vi "Phsae_shift_test(3).vi"() -> ()   [LabVIEW 2017]
uses:
  <vilib>/Analysis/3filter.llb/Filter Passband Type.ctl
  <vilib>/Analysis/3filter.llb/FIR Windowed Filter (DBL).vi
  <vilib>/measure/maspectr.llb/FFT Spectrum (Real-Im) for 1 Chan.vi
  <vilib>/Analysis/NI_AALBase.lvlib
  <vilib>/Analysis/NI_AALPro.lvlib
  <vilib>/measure/NI_MAPro.lvlib
panel:
  out "최대값":dbl
  out "크기":i32
  out "S3 phase spectrum":waveform(dbl)(graph)
  out "SUM signal":waveform(dbl)(graph)
  out "S3 signal":waveform(dbl)(graph)
  out "S2 signal":waveform(dbl)(graph)
  out "S1 signal":waveform(dbl)(graph)
  out "S0 signal":waveform(dbl)(graph)
  out "S3 FFT":waveform(dbl)(graph)
  out "S2 FFT":waveform(dbl)(graph)
  out "S1 FFT":waveform(dbl)(graph)
  out "S0 FFT":waveform(dbl)(graph)
  in  "S3 Carrier Phsae":dbl=270.0
  in  "S2 Carrier Phsae":dbl=180.0
  in  "S1 Carrier Phsae":dbl=90.0
  in  "S0 Carrier Phsae":dbl=90.0
  in  "S3 Phsae":dbl=270.0
  in  "S2 Phsae":dbl=180.0
  in  "S1 Phsae":dbl=90.0
  in  "S0 Phsae":dbl=90.0
  in  "Carrier Frequency(Hz)":dbl=560000.0
  in  "Frequency(Hz)":dbl=600000.0
  in  "Amplitude(Vpeak)":dbl=1.0
  in  "Pulse length(sec)":dbl=0.5
  in  "Sampling frequency(Hz)":dbl=3000000.0
  in  "Delay time.A.1(sec)":dbl=0.5
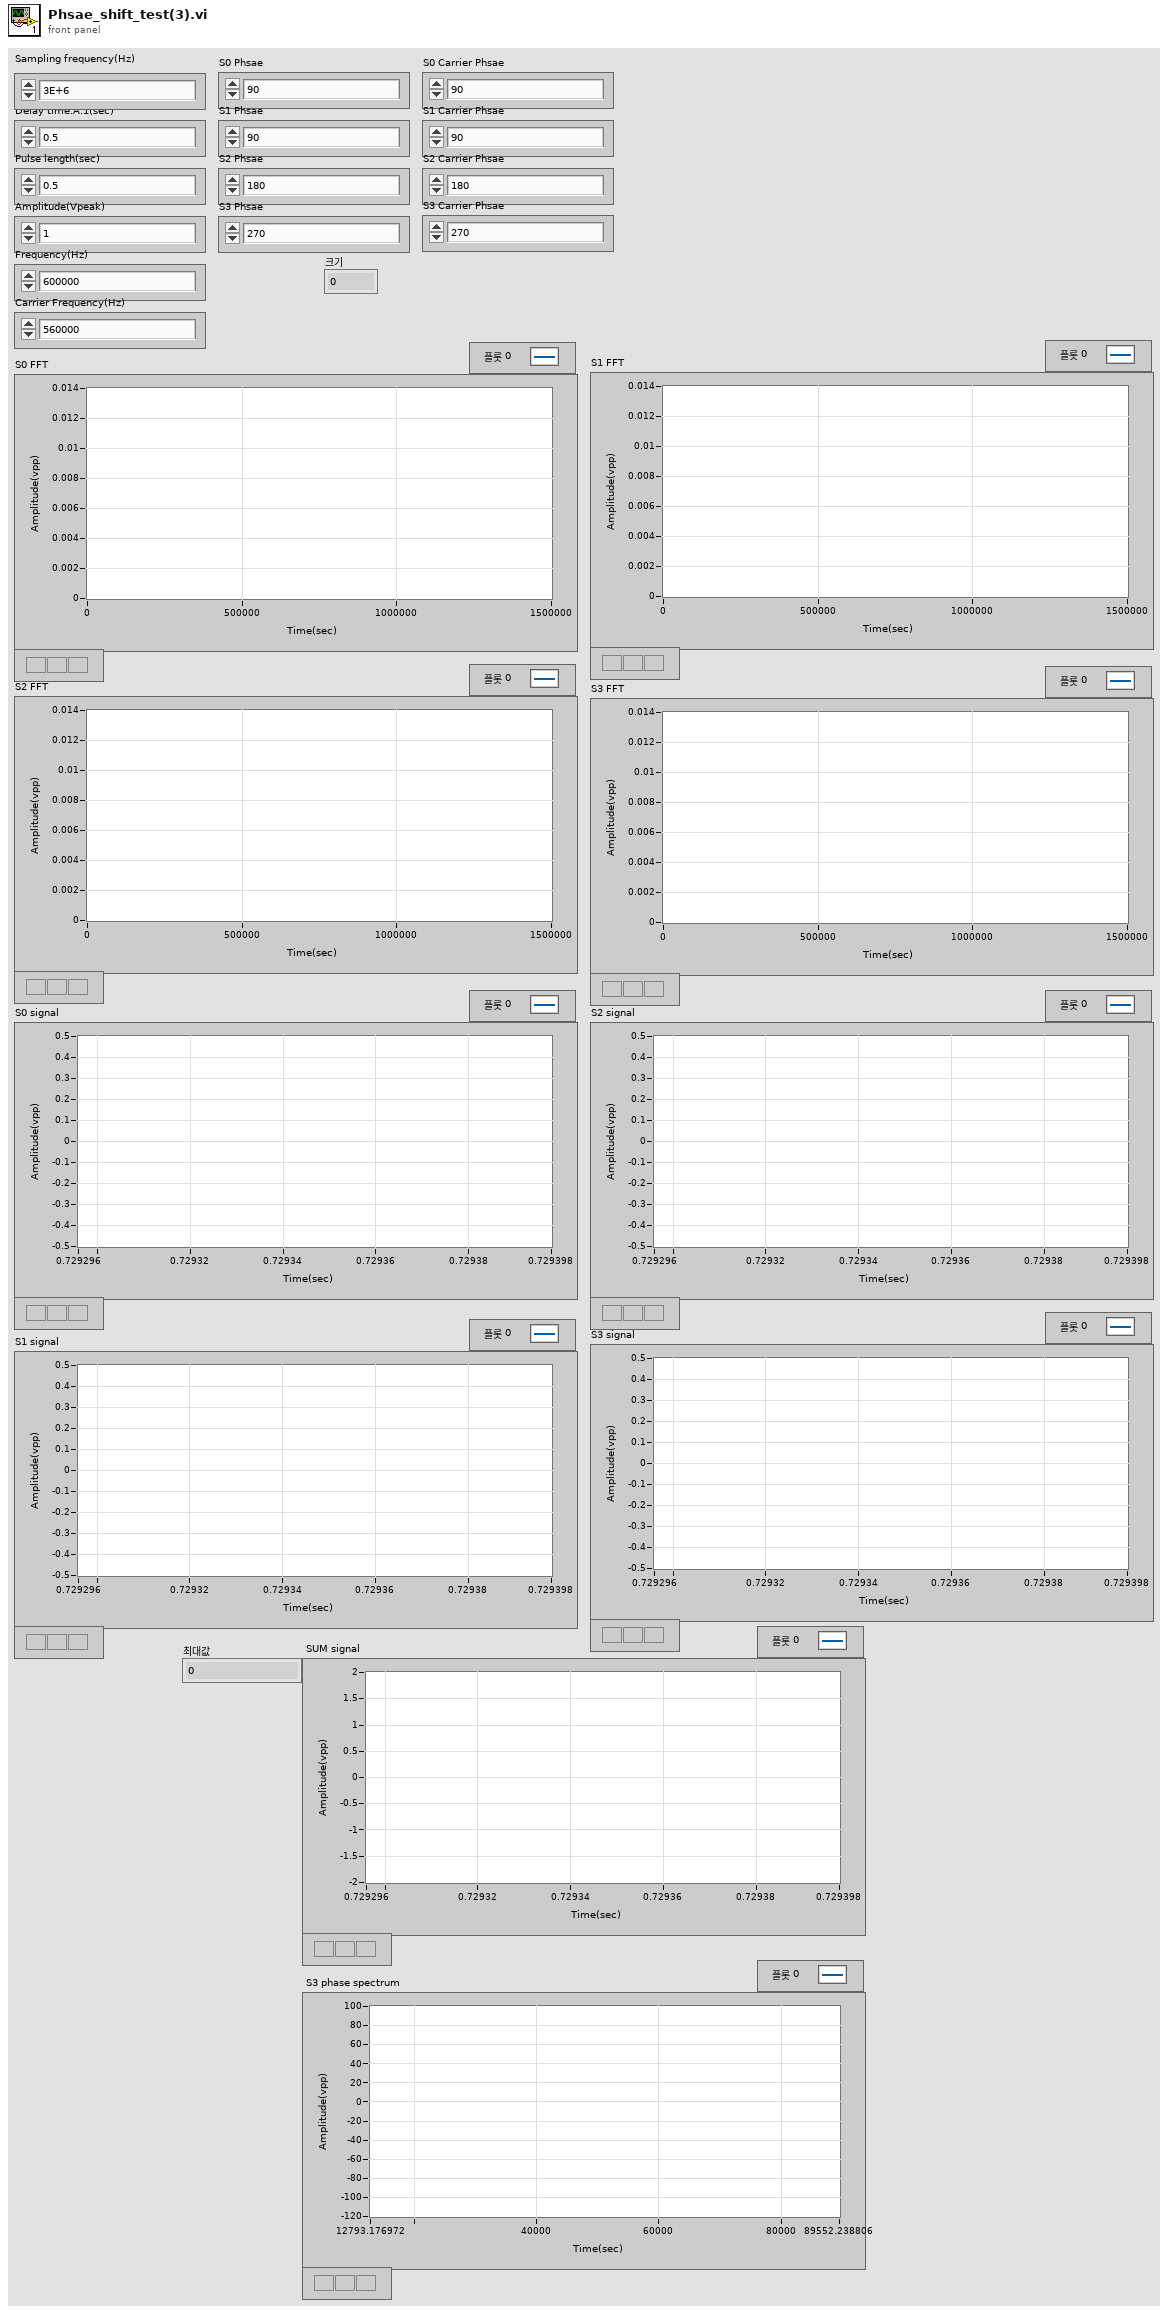
[diagram p1: front panel]
types:
  T1 = typedef "NI_AALBase.lvlib/Filter Passband Type.ctl" = enum32{"Lowpass", "Highpass", "Bandpass", "Bandstop"}
  T2 = cluster{"f0":dbl, "df":dbl, "imaginary part":dbl[]}
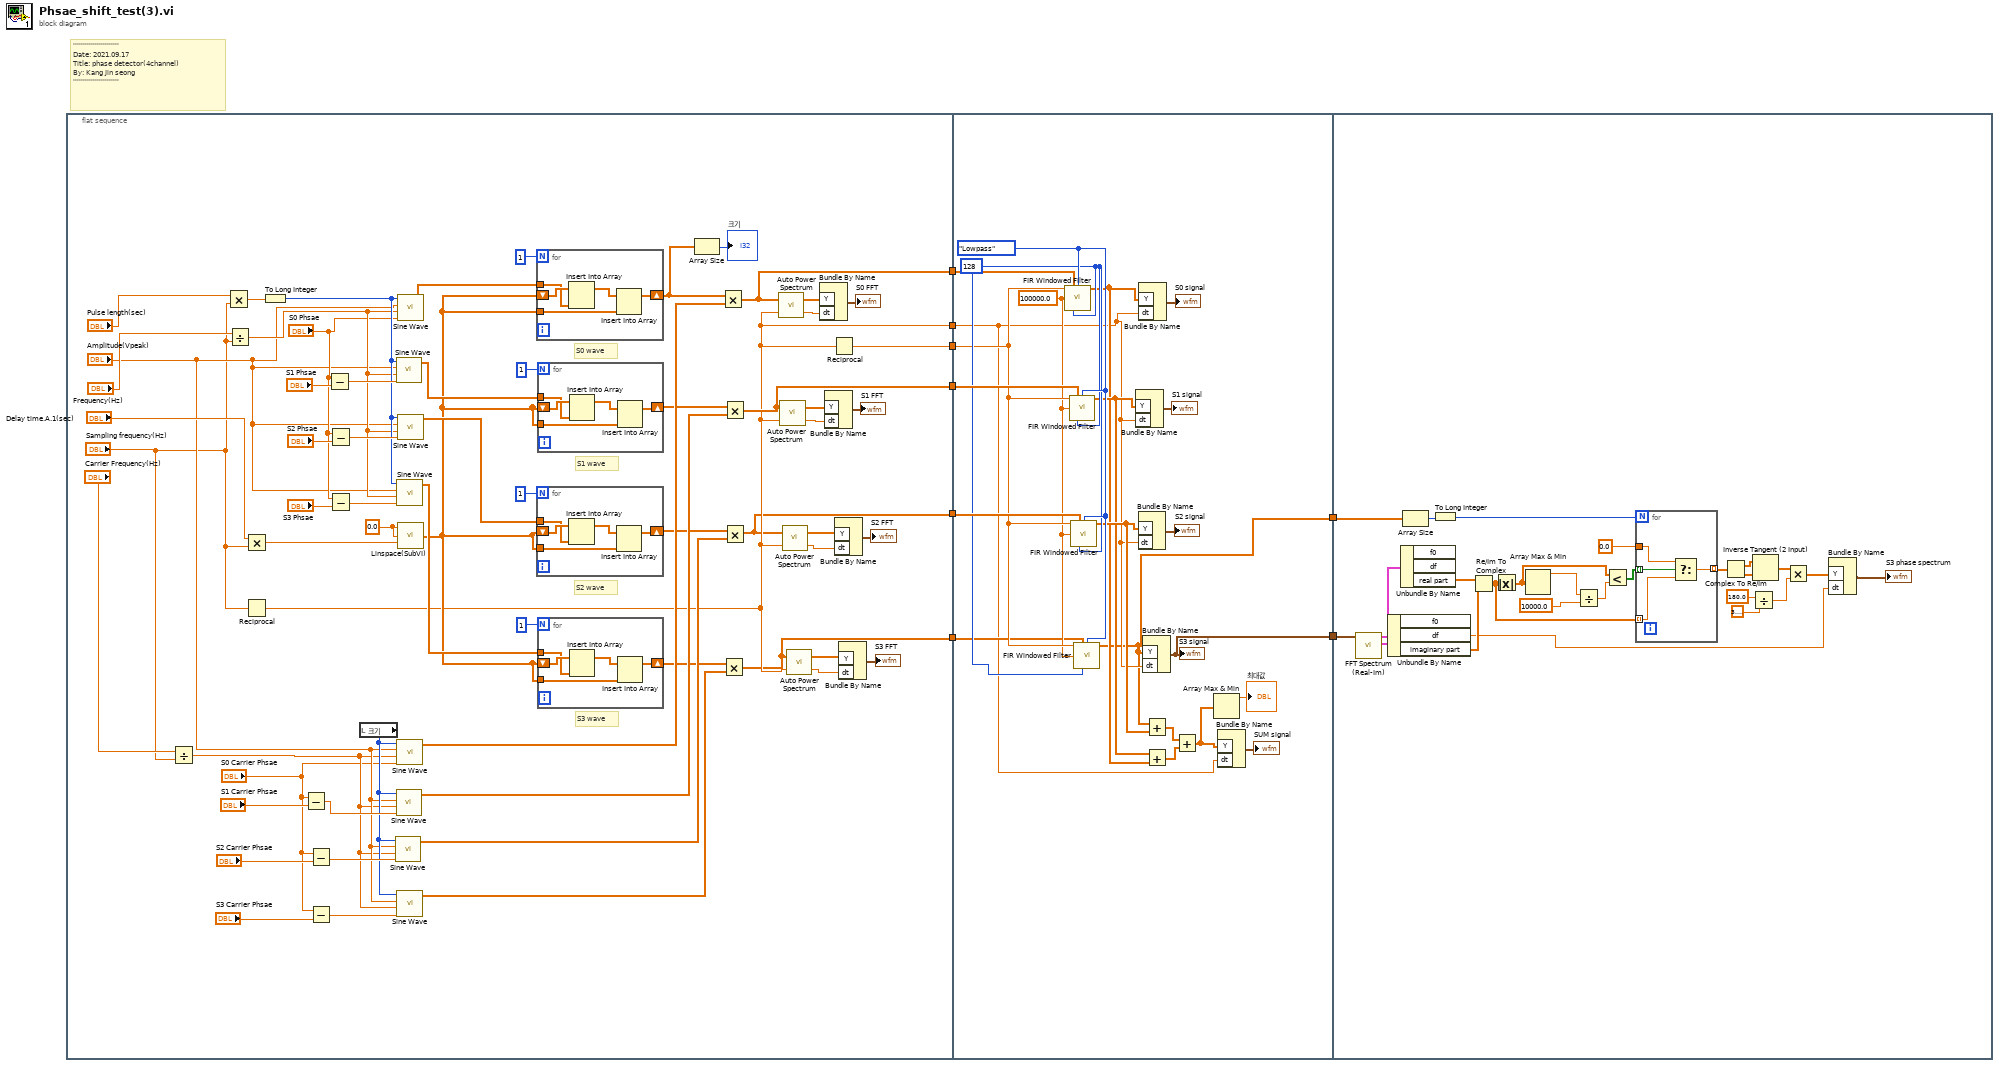
[diagram p0: block diagram]
diagram:
  # "'''''''''''''''''''''''\nDate: 2021.09.17\nTitle: phase detector(4channel)\nBy: Kang Jin seong\n'''''''''''''''''''''''"
  n1 = flat-sequence {
    tunnel: [w18] -> w8
    tunnel: [w17] -> w7
    tunnel: [w16] -> w6
    tunnel: [w13] -> w5
    tunnel: [w12] -> w4
    tunnel: [w11] -> w3
    tunnel: w8 -> [w108]
    tunnel: w7 -> [w113]
    tunnel: w6 -> [w112]
    tunnel: w5 -> [w99]
    tunnel: w4 -> [w111]
    tunnel: w3 -> [w106]
    tunnel: [w95] -> w2
    tunnel: [w94] -> w1
    tunnel: w2 -> [w138]
    tunnel: w1 -> [w131]
    frame #0 {
      w59 = 0.0 ("Start")
      # "S3 wave"
      # "S2 wave"
      # "S1 wave"
      # "S0 wave"
      n2 = Divide(x="Carrier Frequency(Hz)", y="Sampling frequency(Hz)") -> (x/y=w40:dbl)
      n3 = Multiply(x="Pulse length(sec)", y="Sampling frequency(Hz)") -> (x*y=w70:dbl)
      n4 = Divide(x="Frequency(Hz)", y="Sampling frequency(Hz)") -> (x/y=w62:dbl)
      n5 = Multiply(x="Delay time.A.1(sec)", y="Sampling frequency(Hz)") -> (x*y=w57:dbl)
      n6 = Reciprocal(x="Sampling frequency(Hz)") -> (1/x=w13:dbl)
      n7 = To Long Integer(number=w70) -> (32bit integer=w63:i32)
      n8 = Subtract(x="S0 Carrier Phsae", y="S1 Carrier Phsae") -> (x-y=w45:dbl)
      n9 = Subtract(x="S0 Carrier Phsae", y="S2 Carrier Phsae") -> (x-y=w44:dbl)
      n10 = Subtract(x="S0 Carrier Phsae", y="S3 Carrier Phsae") -> (x-y=w39:dbl)
      n11 = Subtract(x="S0 Phsae", y="S1 Phsae") -> (x-y=w67:dbl)
      n12 = Subtract(x="S0 Phsae", y="S2 Phsae") -> (x-y=w64:dbl)
      n13 = Subtract(x="S0 Phsae", y="S3 Phsae") -> (x-y=w61:dbl)
      n14 = local read "크기"() -> (w42:i32)
      n15 = call <vilib>:"Sine Wave.vi"("samples"=w42, "amplitude"="Amplitude(Vpeak)", "frequency"=w40, "phase in"=w44) -> ("sine wave"=w31:dbl[])  [unwired: 1 in, 2 out]
      n16 = call <vilib>:"Sine Wave.vi"("samples"=w63, "amplitude"="Amplitude(Vpeak)", "frequency"=w62, "phase in"=w67) -> ("sine wave"=w53:dbl[])  [unwired: 1 in, 2 out]
      n17 = call <vilib>:"Sine Wave.vi"("samples"=w42, "amplitude"="Amplitude(Vpeak)", "frequency"=w40, "phase in"=w45) -> ("sine wave"=w33:dbl[])  [unwired: 1 in, 2 out]
      n18 = call <vilib>:"Sine Wave.vi"("samples"=w63, "amplitude"="Amplitude(Vpeak)", "frequency"=w62, "phase in"=w61) -> ("sine wave"=w49:dbl[])  [unwired: 1 in, 2 out]
      n19 = call <vilib>:"Sine Wave.vi"("samples"=w42, "amplitude"="Amplitude(Vpeak)", "frequency"=w40, "phase in"="S0 Carrier Phsae") -> ("sine wave"=w36:dbl[])  [unwired: 1 in, 2 out]
      n20 = call <vilib>:"Sine Wave.vi"("samples"=w42, "amplitude"="Amplitude(Vpeak)", "frequency"=w40, "phase in"=w39) -> ("sine wave"=w29:dbl[])  [unwired: 1 in, 2 out]
      n21 = call <vilib>:"Sine Wave.vi"("samples"=w63, "amplitude"="Amplitude(Vpeak)", "frequency"=w62, "phase in"="S0 Phsae") -> ("sine wave"=w55:dbl[])  [unwired: 1 in, 2 out]
      n22 = call <vilib>:"Sine Wave.vi"("samples"=w63, "amplitude"="Amplitude(Vpeak)", "frequency"=w62, "phase in"=w64) -> ("sine wave"=w51:dbl[])  [unwired: 1 in, 2 out]
      n23 = call "Linspace(SubVI).vi"("NumElements"=w57, "End"=w59, "Start"=w59) -> ("Array"=w48:dbl[])
      n24 = for {
        N: 1 -> [_]
        shift-right: [w87] -> w10
        shift-left: w48 -> [w91]
        tunnel: w55 -> [w90]
        tunnel: w48 -> [w88]
        n25 = Insert Into Array(array=w91, new element=w90) -> (w89:dbl[])  [unwired: 1 in]
        n26 = Insert Into Array(array=w89, new element=w88) -> (w87:dbl[])  [unwired: 1 in]
      }
      n27 = for {
        N: 1 -> [_]
        shift-right: [w77] -> w32
        shift-left: w48 -> [w81]
        tunnel: w51 -> [w80]
        tunnel: w48 -> [w78]
        n28 = Insert Into Array(array=w81, new element=w80) -> (w79:dbl[])  [unwired: 1 in]
        n29 = Insert Into Array(array=w79, new element=w78) -> (w77:dbl[])  [unwired: 1 in]
      }
      n30 = for {
        N: 1 -> [_]
        shift-right: [w82] -> w34
        shift-left: w48 -> [w86]
        tunnel: w53 -> [w85]
        tunnel: w48 -> [w83]
        n31 = Insert Into Array(array=w86, new element=w85) -> (w84:dbl[])  [unwired: 1 in]
        n32 = Insert Into Array(array=w84, new element=w83) -> (w82:dbl[])  [unwired: 1 in]
      }
      n33 = for {
        N: 1 -> [_]
        shift-right: [w72] -> w30
        shift-left: w48 -> [w76]
        tunnel: w49 -> [w75]
        tunnel: w48 -> [w73]
        n34 = Insert Into Array(array=w76, new element=w75) -> (w74:dbl[])  [unwired: 1 in]
        n35 = Insert Into Array(array=w74, new element=w73) -> (w72:dbl[])  [unwired: 1 in]
      }
      n36 = Array Size(array=w10) -> (size(s)=→"크기":i32)
      n37 = Multiply(x=w10, y=w36) -> (x*y=w17:dbl[])
      n38 = Multiply(x=w30, y=w29) -> (x*y=w11:dbl[])
      n39 = Multiply(x=w34, y=w33) -> (x*y=w16:dbl[])
      n40 = Multiply(x=w32, y=w31) -> (x*y=w12:dbl[])
      n41 = call <vilib>:"Auto Power Spectrum.vi"("dt"=w13, "Signal (V)"=w17) -> ("df"=w24:dbl, "Power Spectrum (V^2 rms)"=w23:dbl[])
      n42 = call <vilib>:"Auto Power Spectrum.vi"("dt"=w13, "Signal (V)"=w16) -> ("df"=w21:dbl, "Power Spectrum (V^2 rms)"=w22:dbl[])
      n43 = call <vilib>:"Auto Power Spectrum.vi"("dt"=w13, "Signal (V)"=w12) -> ("df"=w20:dbl, "Power Spectrum (V^2 rms)"=w15:dbl[])
      n44 = call <vilib>:"Auto Power Spectrum.vi"("dt"=w13, "Signal (V)"=w11) -> ("df"=w19:dbl, "Power Spectrum (V^2 rms)"=w14:dbl[])
      n45 = Bundle By Name("Y"=w23, "dt"=w24) -> (→"S0 FFT":waveform(dbl))  [unwired: 1 in]
      n46 = Bundle By Name("Y"=w22, "dt"=w21) -> (→"S1 FFT":waveform(dbl))  [unwired: 1 in]
      n47 = Reciprocal(x=w13) -> (1/x=w18:dbl)
      n48 = Bundle By Name("Y"=w15, "dt"=w20) -> (→"S2 FFT":waveform(dbl))  [unwired: 1 in]
      n49 = Bundle By Name("Y"=w14, "dt"=w19) -> (→"S3 FFT":waveform(dbl))  [unwired: 1 in]
    }
    frame #1 {
      w110 = Filter_Passband_Type."Lowpass" ("filter type")
      w109 = 128 ("taps")
      w107 = 100000.0 ("low cutoff freq: fl")
      n50 = call-poly <vilib>:"FIR Windowed Filter.vi"("sampling freq: fs"=w108, "X"=w113, "filter type"=w110, "low cutoff freq: fl"=w107, "taps"=w109) -> ("Filtered X"=w103:dbl[])  [unwired: 9 in, 1 out]
      n51 = call-poly <vilib>:"FIR Windowed Filter.vi"("sampling freq: fs"=w108, "X"=w112, "filter type"=w110, "low cutoff freq: fl"=w107, "taps"=w109) -> ("Filtered X"=w104:dbl[])  [unwired: 9 in, 1 out]
      n52 = call-poly <vilib>:"FIR Windowed Filter.vi"("sampling freq: fs"=w108, "X"=w111, "filter type"=w110, "low cutoff freq: fl"=w107, "taps"=w109) -> ("Filtered X"=w105:dbl[])  [unwired: 9 in, 1 out]
      n53 = call-poly <vilib>:"FIR Windowed Filter.vi"("sampling freq: fs"=w108, "X"=w106, "filter type"=w110, "low cutoff freq: fl"=w107, "taps"=w109) -> ("Filtered X"=w94:dbl[])  [unwired: 9 in, 1 out]
      n54 = Bundle By Name("Y"=w104, "dt"=w99) -> (→"S1 signal":waveform(dbl))  [unwired: 1 in]
      n55 = Bundle By Name("Y"=w105, "dt"=w99) -> (→"S2 signal":waveform(dbl))  [unwired: 1 in]
      n56 = Bundle By Name("Y"=w103, "dt"=w99) -> (→"S0 signal":waveform(dbl))  [unwired: 1 in]
      n57 = Bundle By Name("Y"=w94, "dt"=w99) -> (w95:waveform(dbl))  [unwired: 1 in]
      "S3 signal" <- w95
      n58 = Add(x=w94, y=w105) -> (x+y=w102:dbl[])
      n59 = Add(x=w104, y=w103) -> (x+y=w101:dbl[])
      n60 = Add(x=w102, y=w101) -> (x+y=w93:dbl[])
      n61 = Array Max & Min(array=w93) -> (max value=→"최대값":dbl)  [unwired: 3 out]
      n62 = Bundle By Name("Y"=w93, "dt"=w99) -> (→"SUM signal":waveform(dbl))  [unwired: 1 in]
    }
    frame #2 {
      n63 = call-poly <vilib>:"FFT Spectrum (Real-Im).vi"("time signal"=w138) -> ("imaginary part"=w136:T2, "real part"=w137:cluster{"f0":dbl, "df":dbl, "real part":dbl[]})  [unwired: 6 in, 3 out]
      n64 = Unbundle By Name(w136) -> ("df"=w115:dbl, "imaginary part"=w134:dbl[])  [unwired: 1 out]
      n65 = Unbundle By Name(w137) -> ("real part"=w135:dbl[])  [unwired: 2 out]
      n66 = Array Size(array=w131) -> (size(s)=w130:i32)
      n67 = To Long Integer(number=w130) -> (32bit integer=w129:i32)
      n68 = Re/Im To Complex(1:w134, 2:w135) -> (0:w124:cdb[])
      n69 = Absolute Value(x=w124) -> (abs(x)=w127:dbl[])
      n70 = Array Max & Min(array=w127) -> (max value=w133:dbl)  [unwired: 3 out]
      n71 = Divide(x=w133, y=10000.0) -> (x/y=w128:dbl)
      n72 = Less?(x=w127, y=w128) -> (x < y?=w126:bool[])
      n73 = for {
        N: w129 -> [_]
        tunnel: w126 -> [w142] mode=indexing
        tunnel: 0.0 ("t") -> [w141]
        tunnel: w124 -> [w140] mode=indexing
        tunnel: [w139] -> w117 mode=indexing
        n74 = Select(t=w141, s=w142, f=w140) -> (s? t:f=w139:cdb)
      }
      n75 = Complex To Re/Im(x + iy=w117) -> (x=w119:dbl[], y=w118:dbl[])
      n76 = Divide(x=180.0, y=3.141592653589793) -> (x/y=w121:dbl)
      n77 = Inverse Tangent (2 Input)(1:w118, 2:w119) -> (0:w120:dbl[])
      n78 = Multiply(x=w120, y=w121) -> (x*y=w116:dbl[])
      n79 = Bundle By Name("Y"=w116, "dt"=w115) -> (→"S3 phase spectrum":waveform(dbl))  [unwired: 1 in]
    }
  }
